vi "Initiate Sample Push.vi"(8 "error in (no error)":errorcluster, 9 "Source Storage (None)":T1, 10 "Sample mBar":dbl, 11 "cRIO-CO2 in":refnum<class "cRIO-CO2.lvclass">) -> (0 "error out":errorcluster, 3 "cRIO-CO2 out":refnum<class "cRIO-CO2.lvclass">)   [LabVIEW 2015, in "cRIO-Carbondioxide.lvlib" / "cRIO-CO2.lvlib" / "cRIO-CO2.lvclass"]
uses:
  cRIO-CO2.lvclass
  Controls/Sample Transfer Container Enumerator.ctl
  cRIO-CO2.lvclass/cRIO-CO2.ctl
  Controls/Sample Push State Enumerator.ctl
  cRIO-CO2 Messages/Log Message Msg/Log Message Msg.lvclass/Log Message Msg.ctl
  <vilib>/ActorFramework/Message Enqueuer/Message Enqueuer.lvclass/Message Enqueuer.ctl
  <vilib>/ActorFramework/Message Enqueuer/Enqueue.vi
  State Elapsed Time.vi
  <vilib>/ActorFramework/Message Priority Queue/Priority Enqueue.vi
  cRIO-CO2 Messages/Log Message Msg/Log Message Msg.lvclass
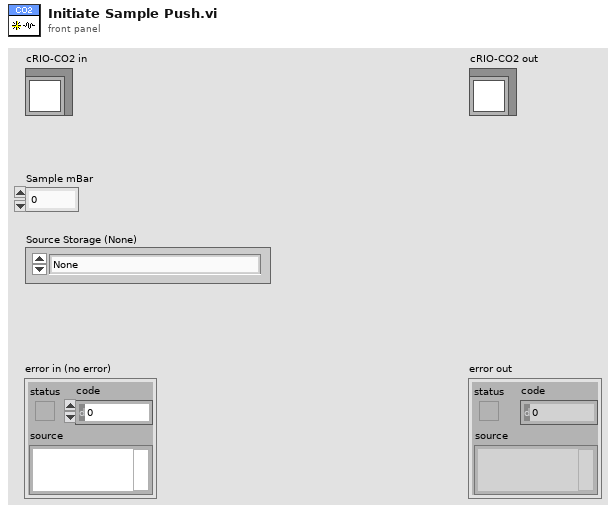
[diagram p1: front panel]
types:
  T1 = typedef "Sample Transfer Container Enumerator.ctl" = enum16{"None", "Sample 1", "Sample 2", "Sample 3", "Sample 4", "Sample 5", "Storage 01", "Storage 02", "Storage 03", "Storage 04", "Storage 05", "Storage 06", "Storage 07", "Storage 08", "Storage 09", "Storage 10", "Storage 11", "Storage 12", "Syringe", "Undefined"}
  T2 = typedef "Sample Push State Enumerator.ctl" = enum16{"Undefined", "Initialize", "Dilute", "Close Transfer Line", "Start Heaters", "Warm Up Syringe", "Ready to Push", "Push", "Initiate Stash", "Stash", "Complete", "Abort", "Idle", "Error"}
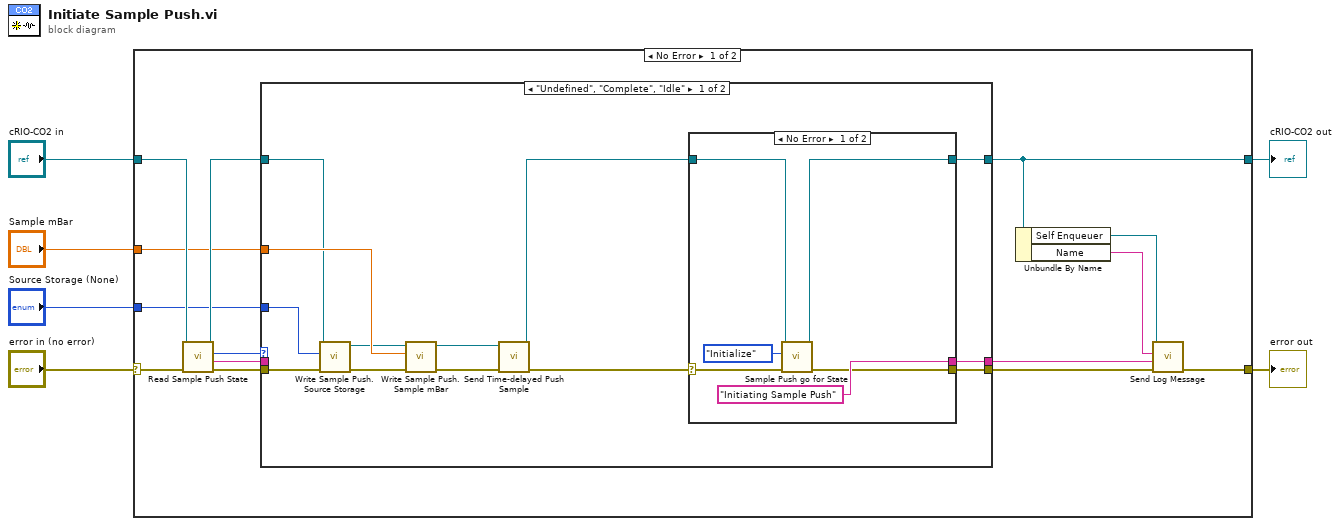
[diagram p0: block diagram]
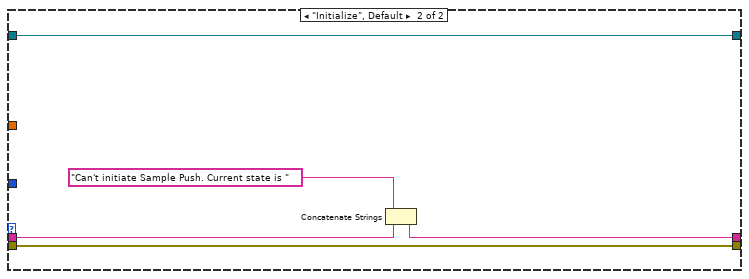
[diagram p3: hidden frame]
diagram:
  n1 = case shown="No Error" "error in (no error)" {
    selector: "error in (no error)" -> [w20 w48]
    tunnel: [w12 w48] -> w5
    tunnel: [w14 w47] -> w3
    tunnel: "cRIO-CO2 in" -> [w19 w47]
    tunnel: "Sample mBar" -> [w8 _]
    tunnel: "Source Storage (None)" -> [w7 _]
    frame No Error {
      n2 = call "Read Sample Push State.vi"("error in (no error)"=w20, "cRIO-CO2 in"=w19) -> ("error out"=w17:errorcluster, 1:"Sample Push State"=w15:string, 2:"Sample Push State"=w18:T2, "cRIO-CO2 out"=w16:refnum<class "cRIO-CO2.lvclass">)  [unwired: 3 in, 3 out]
      n3 = case shown="\"Undefined\", \"Complete\", \"Idle\"" w18 {
        tunnel: w17 -> [w28 w44]
        tunnel: [w32 w46] -> w14
        tunnel: w16 -> [w22 w46]
        tunnel: [w33 w44] -> w13
        tunnel: w15 -> [_ w43]
        tunnel: [w31 w45] -> w10
        tunnel: w8 -> [w25 _]
        tunnel: w7 -> [w24 _]
        frame "Undefined", "Complete", "Idle" {
          n4 = call "Write Sample Push.Source Storage.vi"("error in (no error)"=w28, "Source Storage (None)"=w24, "cRIO-CO2 in"=w22) -> ("error out"=w27:errorcluster, "cRIO-CO2 out"=w23:refnum<class "cRIO-CO2.lvclass">)  [unwired: 7 in]
          n5 = call "Write Sample Push.Sample mBar.vi"("error in (no error)"=w27, "Sample mBar (0)"=w25, "cRIO-CO2 in"=w23) -> ("error out"=w26:errorcluster, "cRIO-CO2 out"=w21:refnum<class "cRIO-CO2.lvclass">)  [unwired: 7 in]
          n6 = call "Send Time-delayed Push Sample.vi"("error in (no error)"=w26, "cRIO-CO2 in"=w21) -> ("error out"=w30:errorcluster, "cRIO-CO2 out"=w29:refnum<class "cRIO-CO2.lvclass">)  [unwired: 8 in]
          n7 = case shown="No Error" w30 {
            selector: w30 -> [w38 w40]
            tunnel: ["Initiating Sample Push" _] -> w31
            tunnel: [w34 w41] -> w32
            tunnel: [w37 w40] -> w33
            tunnel: w29 -> [w36 w41]
            frame No Error {
              n8 = call "Sample Push go for State.vi"("error in (no error)"=w38, "Sample Push State"=Sample_Push_State_Enumerator."Initialize", "cRIO-CO2 in"=w36) -> ("error out"=w37:errorcluster, "cRIO-CO2 out"=w34:refnum<class "cRIO-CO2.lvclass">)  [unwired: 7 in]
            }
            frame Error {
            }
          }
        }
        frame "Initialize", Default {
          n9 = Concatenate Strings("Can't initiate Sample Push. Current state is ", w43) -> (w45:string)
        }
      }
      n10 = Unbundle By Name(w14) -> ("Self Enqueuer"=w11:refnum<class "Message Enqueuer.lvclass">, "Name"=w9:string)
      n11 = call "Send Log Message.vi"("error in (no error)"=w13, "String"=w10, "Source Name"=w9, "Message Enqueuer"=w11) -> ("error out"=w12:errorcluster)  [unwired: 6 in, 1 out]
    }
    frame Error {
    }
  }
  "error out" <- w5
  "cRIO-CO2 out" <- w3
